vi "ObtenerDatosdelatabla.vi"(9 "Column":i32, 10 "Row":i32, 11 "Prueba32 in":refnum<class "Prueba33.lvclass">) -> (3 "Prueba32 out":refnum<class "Prueba33.lvclass">)   [LabVIEW 2019, in "Prueba33.lvclass"]
uses:
  Prueba33.lvclass
  Prueba33.lvclass/Prueba33.ctl
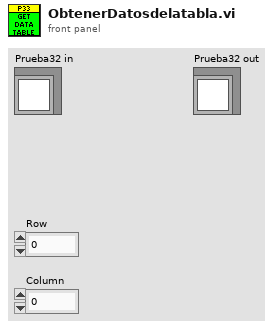
[diagram p1: front panel]
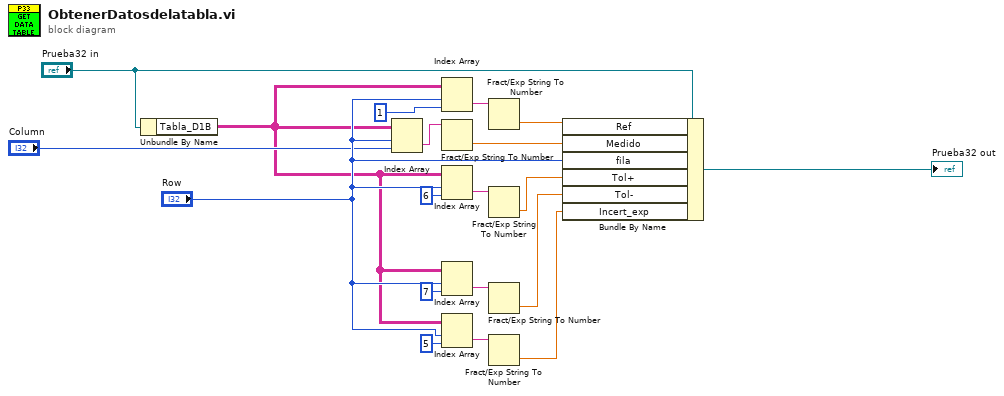
[diagram p0: block diagram]
diagram:
  n1 = Unbundle By Name("Prueba32 in") -> ("Tabla_D1B"=w1:string[][])
  n2 = Index Array(array=w1, index (row)="Row", index (col)="Column") -> (element=w5:string)
  n3 = Index Array(array=w1, index (row)="Row", index (col)=1 ("disabled index (col)")) -> (element=w8:string)
  n4 = Fract/Exp String To Number(string=w5) -> (number=w6:dbl)  [unwired: 3 in, 1 out]
  n5 = Index Array(array=w1, index (row)="Row", index (col)=6 ("disabled index (col)")) -> (element=w10:string)
  n6 = Index Array(array=w1, index (row)="Row", index (col)=7 ("disabled index (col)")) -> (element=w13:string)
  n7 = Index Array(array=w1, index (row)="Row", index (col)=5 ("disabled index (col)")) -> (element=w17:string)
  n8 = Fract/Exp String To Number(string=w8) -> (number=w9:dbl)  [unwired: 3 in, 1 out]
  n9 = Fract/Exp String To Number(string=w10) -> (number=w11:dbl)  [unwired: 3 in, 1 out]
  n10 = Fract/Exp String To Number(string=w13) -> (number=w14:dbl)  [unwired: 3 in, 1 out]
  n11 = Fract/Exp String To Number(string=w17) -> (number=w19:dbl)  [unwired: 3 in, 1 out]
  n12 = Bundle By Name(cluster="Prueba32 in", "Ref"=w9, "Medido"=w6, "fila"="Row", "Tol+"=w11, "Tol-"=w14, "Incert_exp"=w19) -> (→"Prueba32 out":refnum<class "Prueba33.lvclass">)
